vi "Msg To Caller.vi"(9 "Priority Msg?":bool, 10 "Msg":refnum<class "Msg.lvclass">, 11 "jettl in":refnum<class "jettl.lvclass">) -> (0 "error out":errorcluster)   [LabVIEW 2021, in "jettl.lvlib" / "jettl.lvclass"]
uses:
  jettl.lvclass
  Actor/Msg/Msg.lvclass
  jettl.lvclass/jettl.ctl
  jettl.lvlib
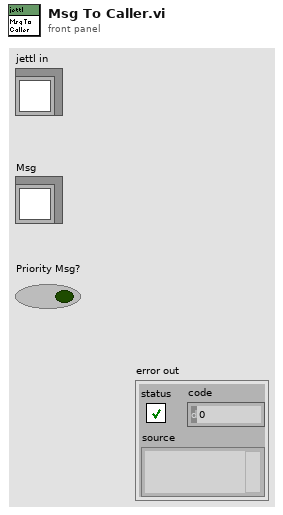
[diagram p1: front panel]
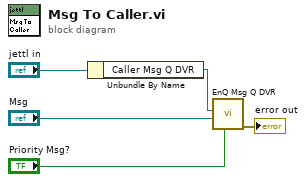
[diagram p0: block diagram]
diagram:
  n1 = Unbundle By Name("jettl in") -> ("Caller Msg Q DVR"=w5:refnum<data-value>)
  n2 = call "EnQ Msg Q DVR.vi"("Priority Msg?"="Priority Msg?", "Msg"="Msg", "Msg Q DVR"=w5) -> ("error out"=→"error out":errorcluster)  [unwired: 8 in]
